vi "FIFO Core U128 - FPGA RAM.vi"(0 "input data":cluster{"high":u64, "low":u64}, 1 "reset":bool, 2 "fifo memory":refnum<k21>, 3 "fifo depth":u8(ring)=10 items=["4"=2, "8"=3, "16"=4, "32"=5, "64"=6, "128"=7, "256"=8, "512"=9, "1024"=10, "2048"=11, "4096"=12, "8192"=13, "16384"=14, "32768"=15, "65536"=16], 9 "input valid":bool, 12 "ready for output":bool=TRUE) -> (4 "output data":cluster{"high":u64, "low":u64}, 6 "state":T1, 10 "output valid":bool, 14 "ready for input":bool)   [LabVIEW 2011, in "FIFO.lvlib"]
uses:
  <instrlib>/RF-RIO/FIFO/FIFO/FPGA/FIFO.lvlib
  <instrlib>/RF-RIO/FIFO/FIFO/FPGA/Public/FIFO State.ctl
  <vilib>/rvi/DataTransferAndStorage/Container/Common/niFpgaContainerExecOnDevCompGetState.vi
  <vilib>/rvi/Memory/Memory_Emulation/niFpgaMemoryEmulationValidateCache.vi
  <vilib>/rvi/DataTransferAndStorage/Container/Common/niFpgaContainerGetUniqueNameForEmu.vi
  <vilib>/rvi/Memory/Memory_Emulation/nirvimemoryEmulationManagerCache_InsertValue.vi
  <vilib>/Utility/error.llb/Clear Errors.vi
  <vilib>/rvi/Memory/Memory_Emulation/nirvimemoryEmulationManagerCache_GetValue.vi
  <vilib>/rvi/Memory/Memory_Emulation/nirvimemoryEmulationManagerCache_SetValue.vi
  <vilib>/rvi/DataTransferAndStorage/Container/XNode/niFpgaContainer.xnode
  <vilib>/rvi/Memory/Memory_Emulation/niFpgaMemoryEmulationRefIn.vi
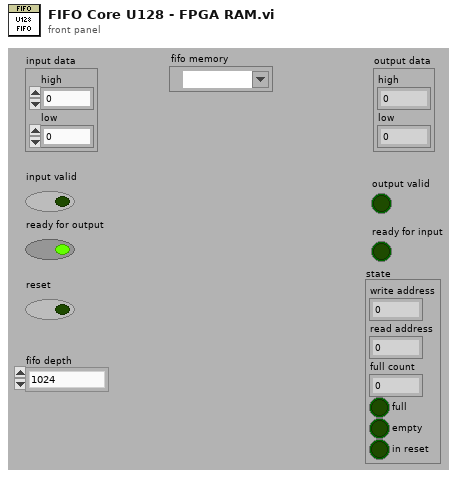
[diagram p1: front panel]
types:
  T1 = typedef "FIFO.lvlib/FIFO State.ctl" = cluster{"write address":u32, "read address":u32, "full count":u32, "full":bool, "empty":bool, "in reset":bool}
  T2 = typedef "FIFO.lvlib/FIFO State - 16-bit Address.ctl" = cluster{"write address":u16, "read address":u16, "full count":u16, "full":bool, "empty":bool}
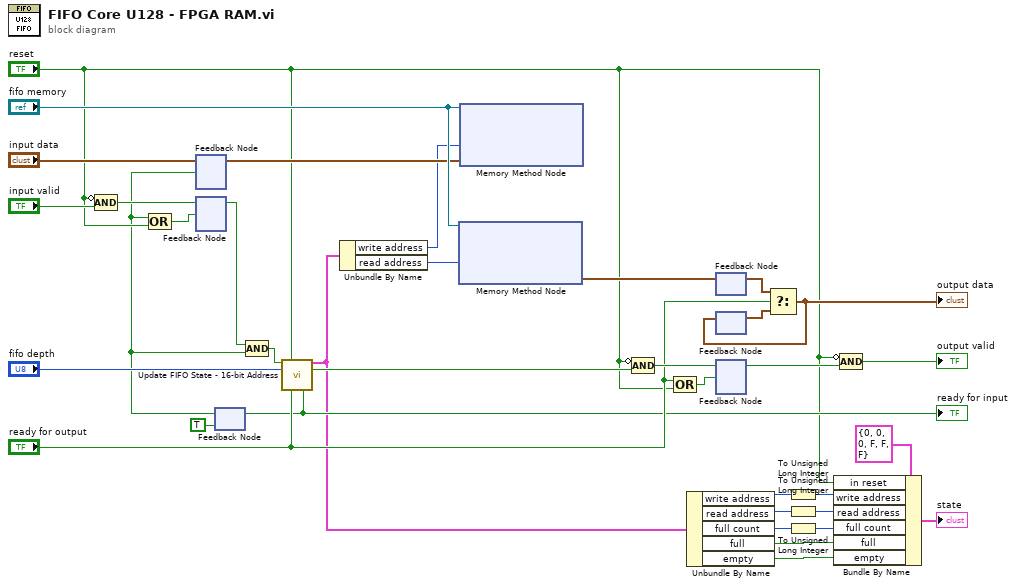
[diagram p0: block diagram]
diagram:
  n1 = Compound Arithmetic op=AND(invert "reset", "input valid") -> (w26:bool)
  n2 = feedback #1() -> (w30:cluster{"high":u64, "low":u64})  [unwired: 1 in]
  n3 = feedback #2() -> (w4:bool)  [unwired: 1 in]
  n4 = feedback #3(TRUE ("ready for write")) -> (w3:bool)
  n5 = Compound Arithmetic op=OR(w3, "reset") -> (w25:bool)
  n6 = feedback-in #1("input data", w3) -> ()
  n7 = feedback-in #2(w26, w25) -> ()
  n8 = Compound Arithmetic op=AND(w4, w3) -> (w2:bool)
  n9 = call <instrlib>:"Update FIFO State - 16-bit Address.vi"("issue write"=w2, "reset"="reset", "fifo depth"="fifo depth", "ready for read request"="ready for output") -> ("state"=w5:T2, "issue read request"=w19:bool, "ready for write"=w17:bool)  [unwired: 9 in]
  "ready for input" <- w17
  n10 = feedback-in #3(w17) -> ()
  n11 = Unbundle By Name(w5) -> ("write address"=w29:u16, "read address"=w28:u16)
  n12 = xnode ("Memory Method Node")("Address"=w28, "Memory In"="fifo memory") -> ("Data"=w24:cluster{"high":u64, "low":u64})  [unwired: 1 out]
  n13 = xnode ("Memory Method Node")("Address"=w29, "Data"=w30, "Memory In"="fifo memory") -> ()  [unwired: 1 out]
  n14 = Compound Arithmetic op=AND(invert "reset", w19) -> (w33:bool)
  n15 = Compound Arithmetic op=OR("ready for output", "reset") -> (w31:bool)
  n16 = Unbundle By Name(w5) -> ("write address"=w15:u16, "read address"=w14:u16, "full count"=w13:u16, "full"=w12:bool, "empty"=w11:bool)
  n17 = feedback #4() -> (w23:cluster{"high":u64, "low":u64})  [unwired: 1 in]
  n18 = feedback-in #4(w24) -> ()
  n19 = feedback #5() -> (w22:cluster{"high":u64, "low":u64})  [unwired: 1 in]
  n20 = feedback #6() -> (w32:bool)  [unwired: 1 in]
  n21 = feedback-in #6(w33, w31) -> ()
  n22 = Select(t=w23, s="ready for output", f=w22) -> (s? t:f=w21:cluster{"high":u64, "low":u64})
  "output data" <- w21
  n23 = feedback-in #5(w21) -> ()
  n24 = To Unsigned Long Integer(number=w15) -> (unsigned 32bit integer=w8:u32)
  n25 = To Unsigned Long Integer(number=w14) -> (unsigned 32bit integer=w7:u32)
  n26 = To Unsigned Long Integer(number=w13) -> (unsigned 32bit integer=w6:u32)
  n27 = Bundle By Name(cluster=T1 {"write address"=0, "read address"=0, "full count"=0, "full"=FALSE, "empty"=FALSE, "in reset"=FALSE} ("state"), "in reset"="reset", "write address"=w8, "read address"=w7, "full count"=w6, "full"=w12, "empty"=w11) -> (→"state":T1)
  n28 = Compound Arithmetic op=AND(invert "reset", w32) -> (→"output valid":bool)
